vi "Set DDG External Output Polarity.vi"(10 "uiPolarity":u32, 11 "uiIndex":u32) -> (3 "function return":u32)   [LabVIEW 2018, in "AndorSDK.lvlib"]
doc: "EXPNETTYPE unsigned int WINAPI SetDDGExternalOutputPolarity(at_u32 uiIndex, at_u32 uiPolarity);"
uses:
  AndorSDK.lvlib
  ATMCD32D.dll
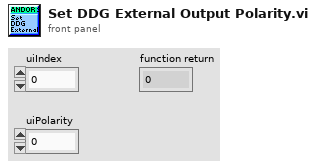
[diagram p1: front panel]
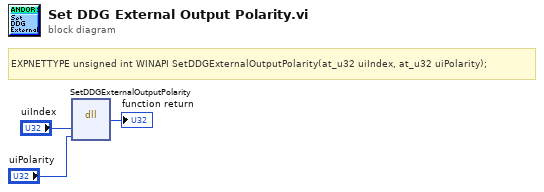
[diagram p0: block diagram]
diagram:
  # "EXPNETTYPE unsigned int WINAPI SetDDGExternalOutputPolarity(at_u32 uiIndex, at_u32 uiPolarity);"
  n1 = dll-call lib="PTH2babs E\nPersönliches02 - Arbeit03-HiwijobsLabviewCodelibANDOR\tAndor SDK\nATMCD32D.*" fn="SetDDGExternalOutputPolarity"("uiIndex"="uiIndex", "uiPolarity"="uiPolarity") -> (→"function return":u32)  [unwired: 5 in, 2 out]
